vi "Status Digital Out.vi"(0 "VISA resource name":refnum<visa-resource-name>, 11 "error in (no error)":errorcluster) -> (4 "VISA resource name out":refnum<visa-resource-name>, 6 "Digital Output Mode":u16(ring) items=["Off", "Alarms", "Scanner", "Manual"], 8 "Digital Input Status":dbl min=0.0 max=63.0 step=1.0, 10 "Manual Output Setting":dbl min=0.0 max=31.0 step=1.0, 14 "Digital Output Status":dbl min=0.0 max=31.0 step=1.0, 15 "error out":errorcluster)   [LabVIEW 2025, in "Lake Shore Cryotronics 340.lvlib"]
doc: "This VI indicates the digital I/O settings and status."
uses:
  Lake Shore Cryotronics 340.lvlib
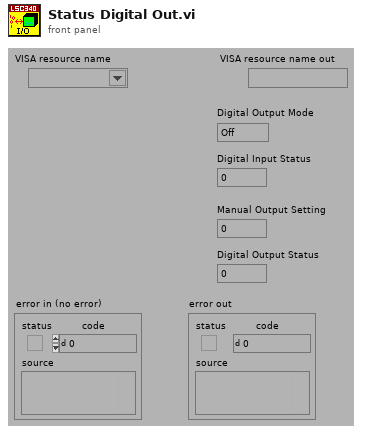
[diagram p1: front panel]
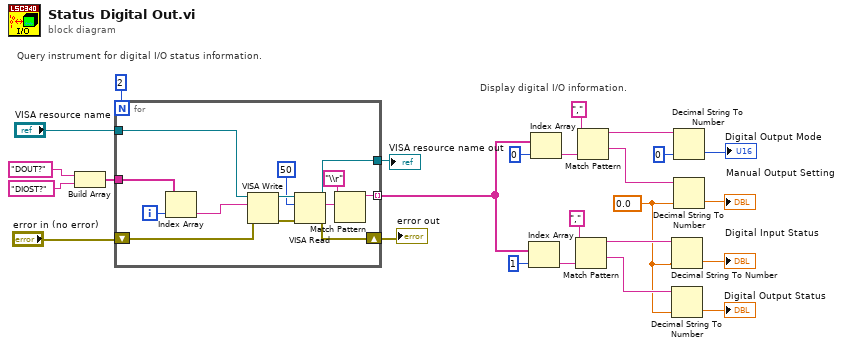
[diagram p0: block diagram]
diagram:
  w1 = 0.0 ("default (0L)")
  # "Query instrument for digital I/O status information."
  # "Display digital I/O information."
  n1 = Build Array("DOUT?", "DIOST?") -> (w10:string[])
  n2 = for {
    N: 2 -> [_]
    tunnel: w10 -> [w34]
    shift-right: [w31] -> w5
    shift-left: "error in (no error)" -> [w32]
    tunnel: [w30] -> w4
    tunnel: [w28] -> w3 mode=indexing
    tunnel: "VISA resource name" -> [w27]
    i -> [w33]
    n3 = Index Array(array=w34, index=w33) -> (element=w26:string)
    n4 = VISA Write(VISA resource name=w27, write buffer=w26, error in (no error)=w32) -> (VISA resource name out=w38:refnum<visa-resource-name>, error out=w37:errorcluster)  [unwired: 1 out]
    n5 = VISA Read(VISA resource name=w38, byte count=50, error in (no error)=w37) -> (VISA resource name out=w30:refnum<visa-resource-name>, read buffer=w35:string, error out=w31:errorcluster)  [unwired: 1 out]
    n6 = Match Pattern(string=w35, regular expression="\\r") -> (before substring=w28:string)  [unwired: 1 in, 3 out]
  }
  "error out" <- w5
  "VISA resource name out" <- w4
  n7 = Index Array(array=w3, index=1) -> (element=w22:string)
  n8 = Index Array(array=w3, index=0) -> (element=w13:string)
  n9 = Match Pattern(string=w22, regular expression=",") -> (before substring=w20:string, after substring=w19:string)  [unwired: 1 in, 2 out]
  n10 = Match Pattern(string=w13, regular expression=",") -> (before substring=w15:string, after substring=w16:string)  [unwired: 1 in, 2 out]
  n11 = Decimal String To Number(string=w20, default (0L)=w1) -> (number=→"Digital Input Status":dbl)  [unwired: 1 in, 1 out]
  n12 = Decimal String To Number(string=w19, default (0L)=w1) -> (number=→"Digital Output Status":dbl)  [unwired: 1 in, 1 out]
  n13 = Decimal String To Number(string=w15, default (0L)=u16 0) -> (number=→"Digital Output Mode":u16)  [unwired: 1 in, 1 out]
  n14 = Decimal String To Number(string=w16, default (0L)=w1) -> (number=→"Manual Output Setting":dbl)  [unwired: 1 in, 1 out]
